vi "De-spiked_Stats.vi"(0 "Raw Signal":dbl[](array[numeric]), 1 "No of st dev to chop at":dbl=6.0) -> (2 "mean":dbl format="%0.2f", 3 "standard deviation":dbl format="%0.2f", 4 "variance":dbl format="%0.2f")   [LabVIEW 2014]
uses:
  <vilib>/Analysis/NI_AALBase.lvlib
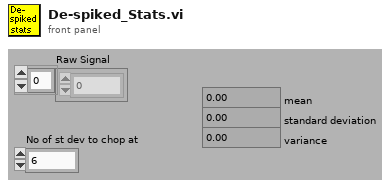
[diagram p1: front panel]
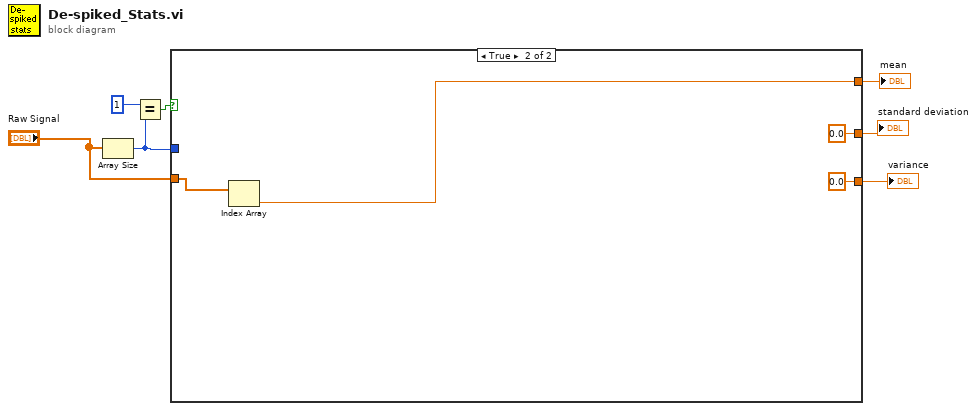
[diagram p0: block diagram]
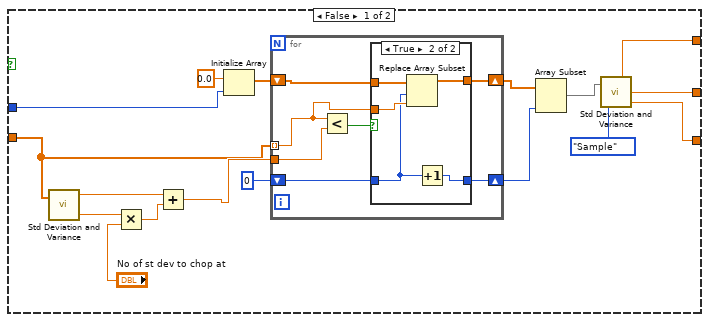
[diagram p2: hidden frame]
diagram:
  n1 = Array Size(array="Raw Signal") -> (size(s)=w3:i32)
  n2 = Equal?(x=1, y=w3) -> (x = y?=w2:bool)
  n3 = case shown="True" w2 {
    tunnel: w3 -> [w24 _]
    tunnel: "Raw Signal" -> [w14 w42]
    tunnel: [w11 w41] -> w6
    tunnel: [w10 0.0 ("standard deviation")] -> w5
    tunnel: [w9 0.0 ("variance")] -> w4
    frame False {
      n4 = call <vilib>:"Std Deviation and Variance.vi"("X"=w14) -> ("mean"=w20:dbl, "standard deviation"=w19:dbl)  [unwired: 1 in, 1 out]
      n5 = Multiply(x=w19, y="No of st dev to chop at") -> (x*y=w18:dbl)
      n6 = Add(x=w20, y=w18) -> (x+y=w17:dbl)
      n7 = Initialize Array(0.0 ("element"), w24) -> (w22:dbl[])
      n8 = for {
        shift-right: [w30] -> w16
        shift-left: w22 -> [w31]
        shift-right: [w25] -> w15
        shift-left: 0 -> [w26]
        tunnel: w17 -> [w29]
        tunnel: w14 -> [w27] mode=indexing
        n9 = Less?(x=w27, y=w29) -> (x < y?=w28:bool)
        n10 = case shown="True" w28 {
          tunnel: w31 -> [w32 w38]
          tunnel: [w32 w37] -> w30
          tunnel: w27 -> [_ w36]
          tunnel: w26 -> [w33 w35]
          tunnel: [w33 w34] -> w25
          frame False {
          }
          frame True {
            n11 = Replace Array Subset(array=w38, new element=w36, index=w35) -> (w37:dbl[])
            n12 = Increment(x=w35) -> (x+1=w34:i32)
          }
        }
      }
      n13 = Array Subset(array=w16, length=w15) -> (w13:dbl[])  [unwired: 1 in]
      n14 = call <vilib>:"Std Deviation and Variance.vi"("X"=w13, "Weighting (Sample)"=enum16{"Sample", "Population"}."Sample") -> ("mean"=w11:dbl, "standard deviation"=w10:dbl, "variance"=w9:dbl)
    }
    frame True {
      n15 = Index Array(array=w42) -> (element=w41:dbl)  [unwired: 1 in]
    }
  }
  "mean" <- w6
  "standard deviation" <- w5
  "variance" <- w4
